vi "get_value.vi"(8 "error in (no error)":errorcluster, 11 "StringLiteral in":refnum<class "StringLiteral.lvclass">) -> (0 "error out":errorcluster, 2 "value":string, 3 "StringLiteral out":refnum<class "StringLiteral.lvclass">)   [LabVIEW 2020, in "mlir.lvlib" / "StringLiteral.lvclass"]
uses:
  StringLiteral.lvclass
  StringLiteral.lvclass/StringLiteral.ctl
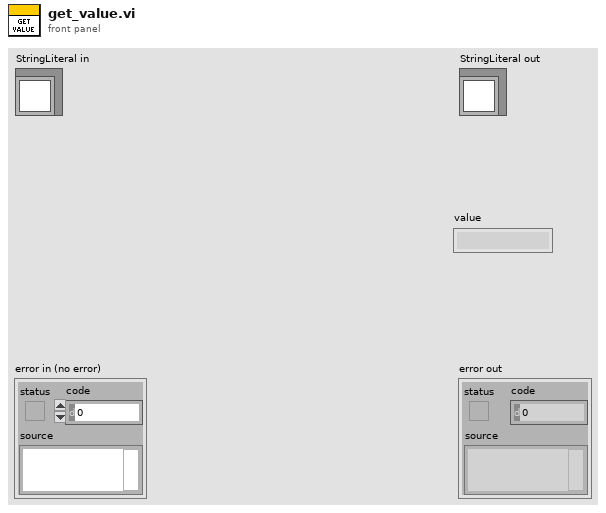
[diagram p1: front panel]
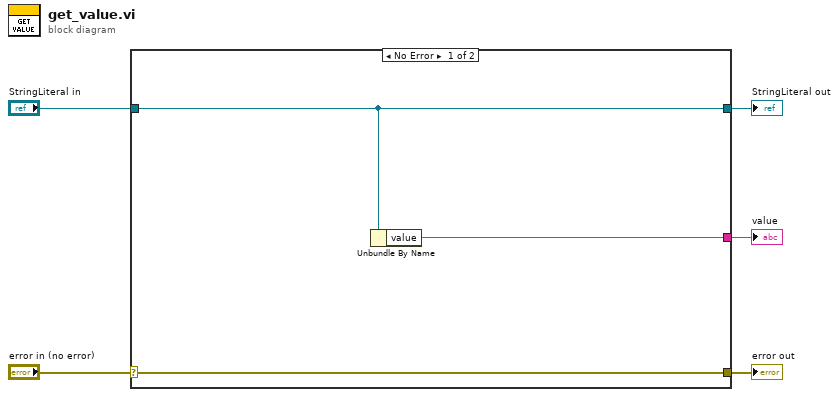
[diagram p0: block diagram]
diagram:
  n1 = case shown="No Error" "error in (no error)" {
    selector: "error in (no error)" -> [w8 w10]
    tunnel: [w8 w10] -> w4
    tunnel: [w7 w9] -> w2
    tunnel: "StringLiteral in" -> [w7 w9]
    tunnel: [w6 _] -> w1
    frame No Error {
      n2 = Unbundle By Name(w7) -> ("value"=w6:string)
    }
    frame Error {
    }
  }
  "error out" <- w4
  "StringLiteral out" <- w2
  "value" <- w1
